vi "License Keya.vi"() -> ()   [LabVIEW 2022 SP3]
panel:
  out "String":string
  in  "Tab Control":enum32{"Page 2"}(tab)
  out "Boolean 4":bool
  out "Boolean 3":bool
  out "Boolean2":bool
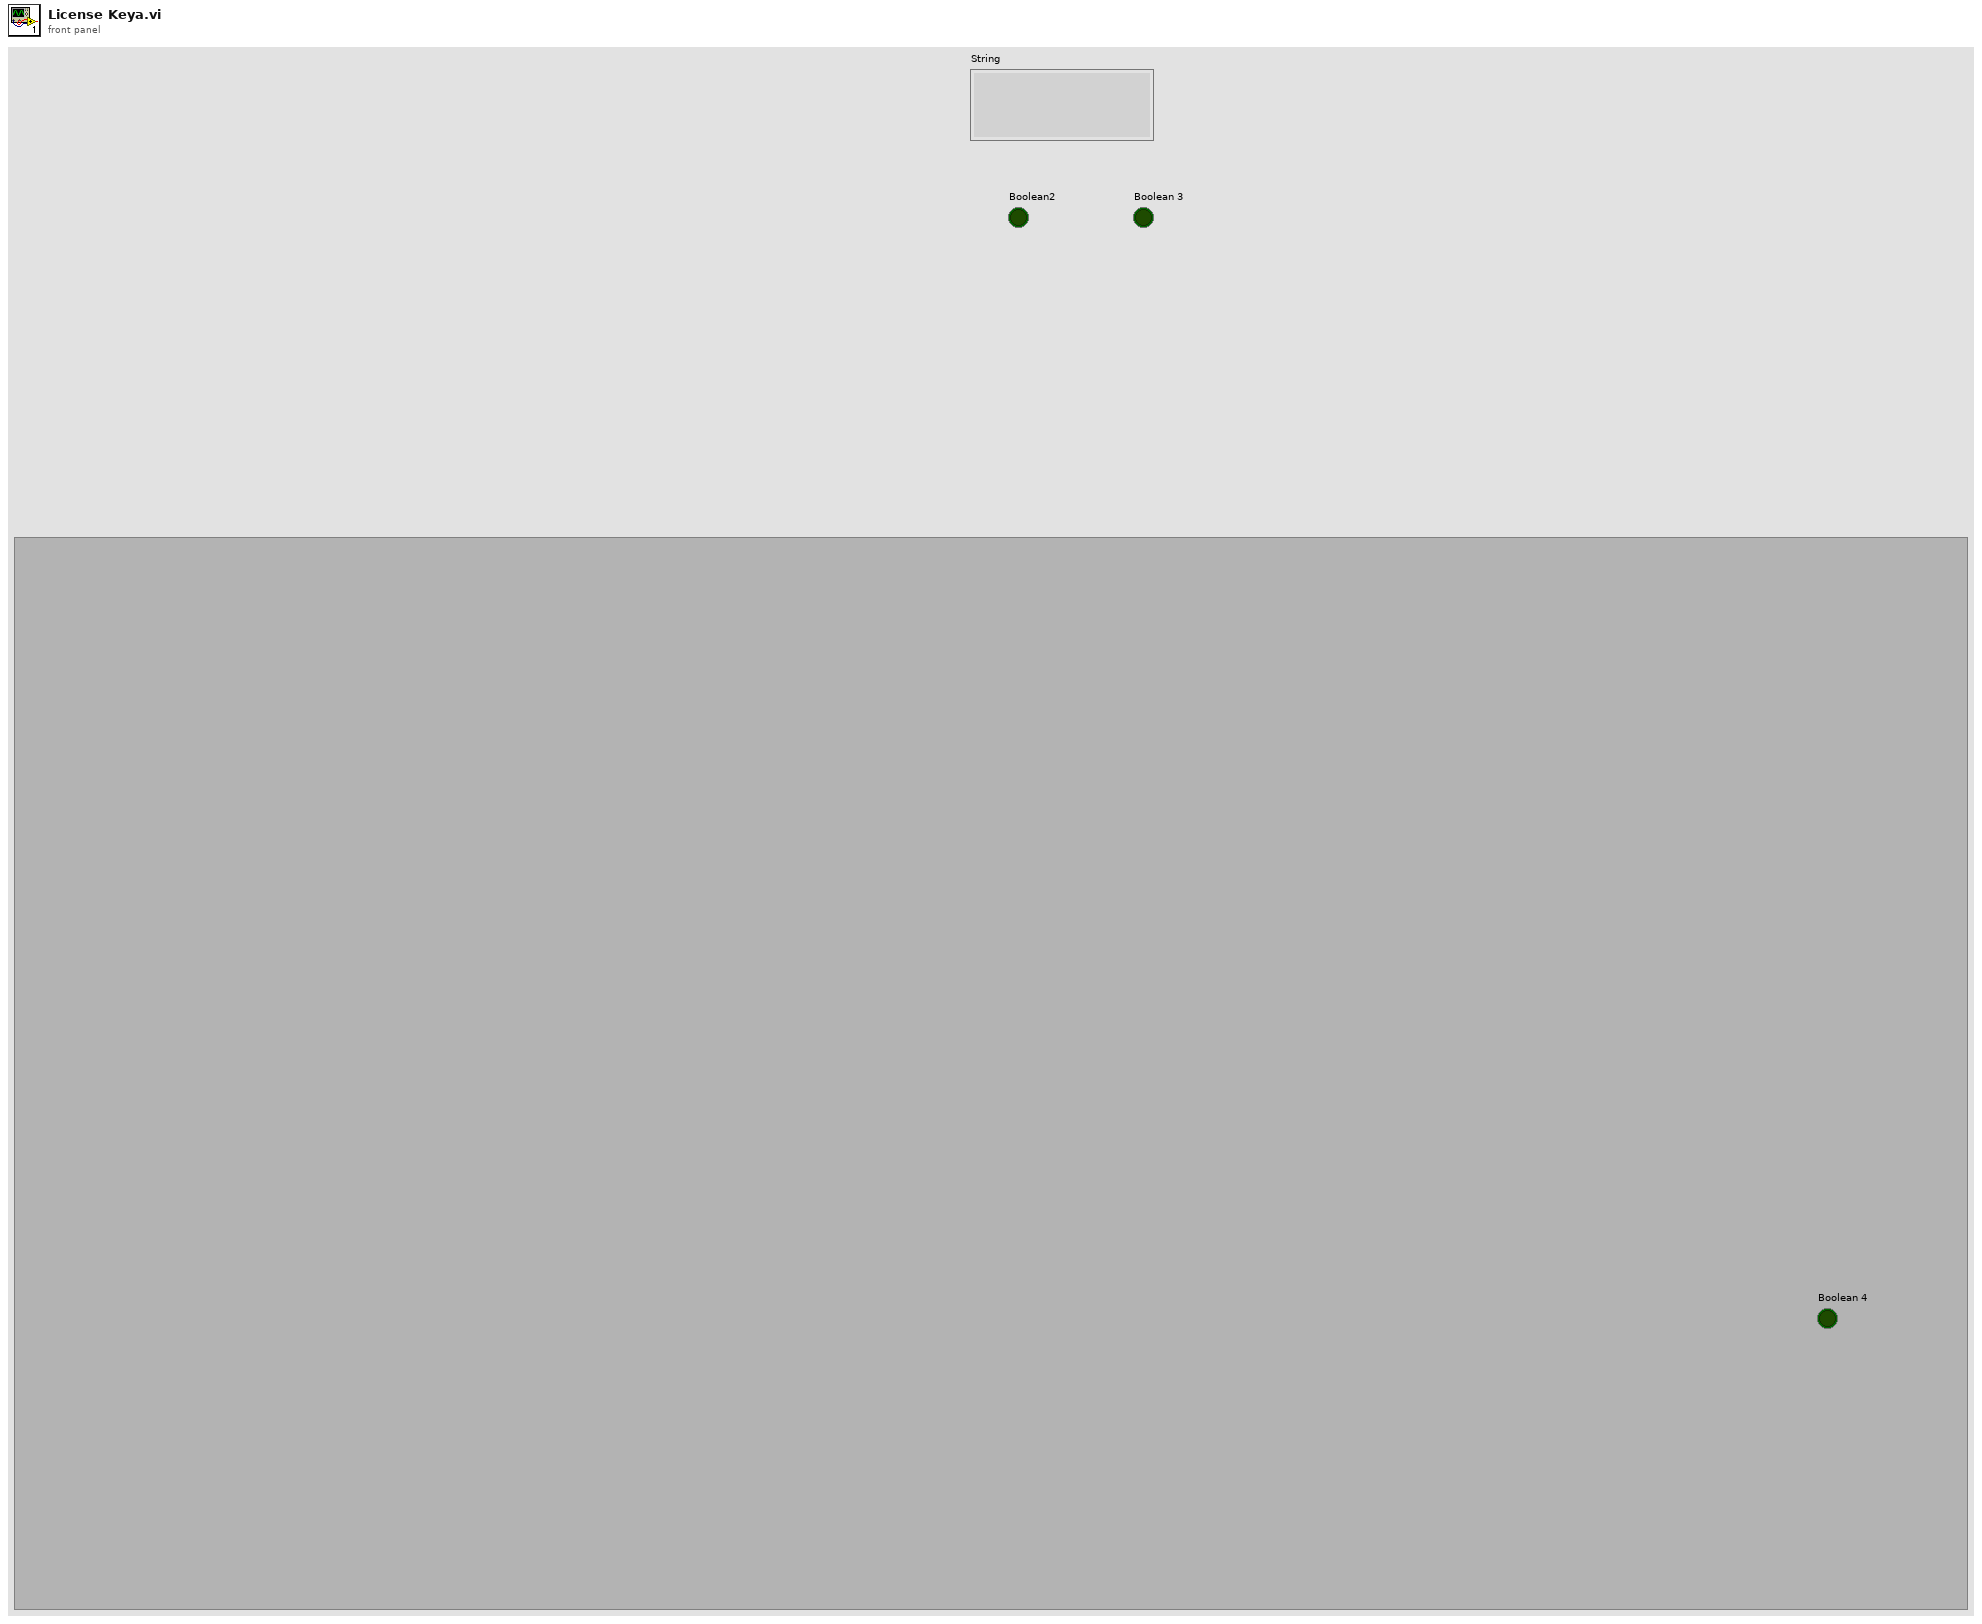
[diagram p1: front panel]
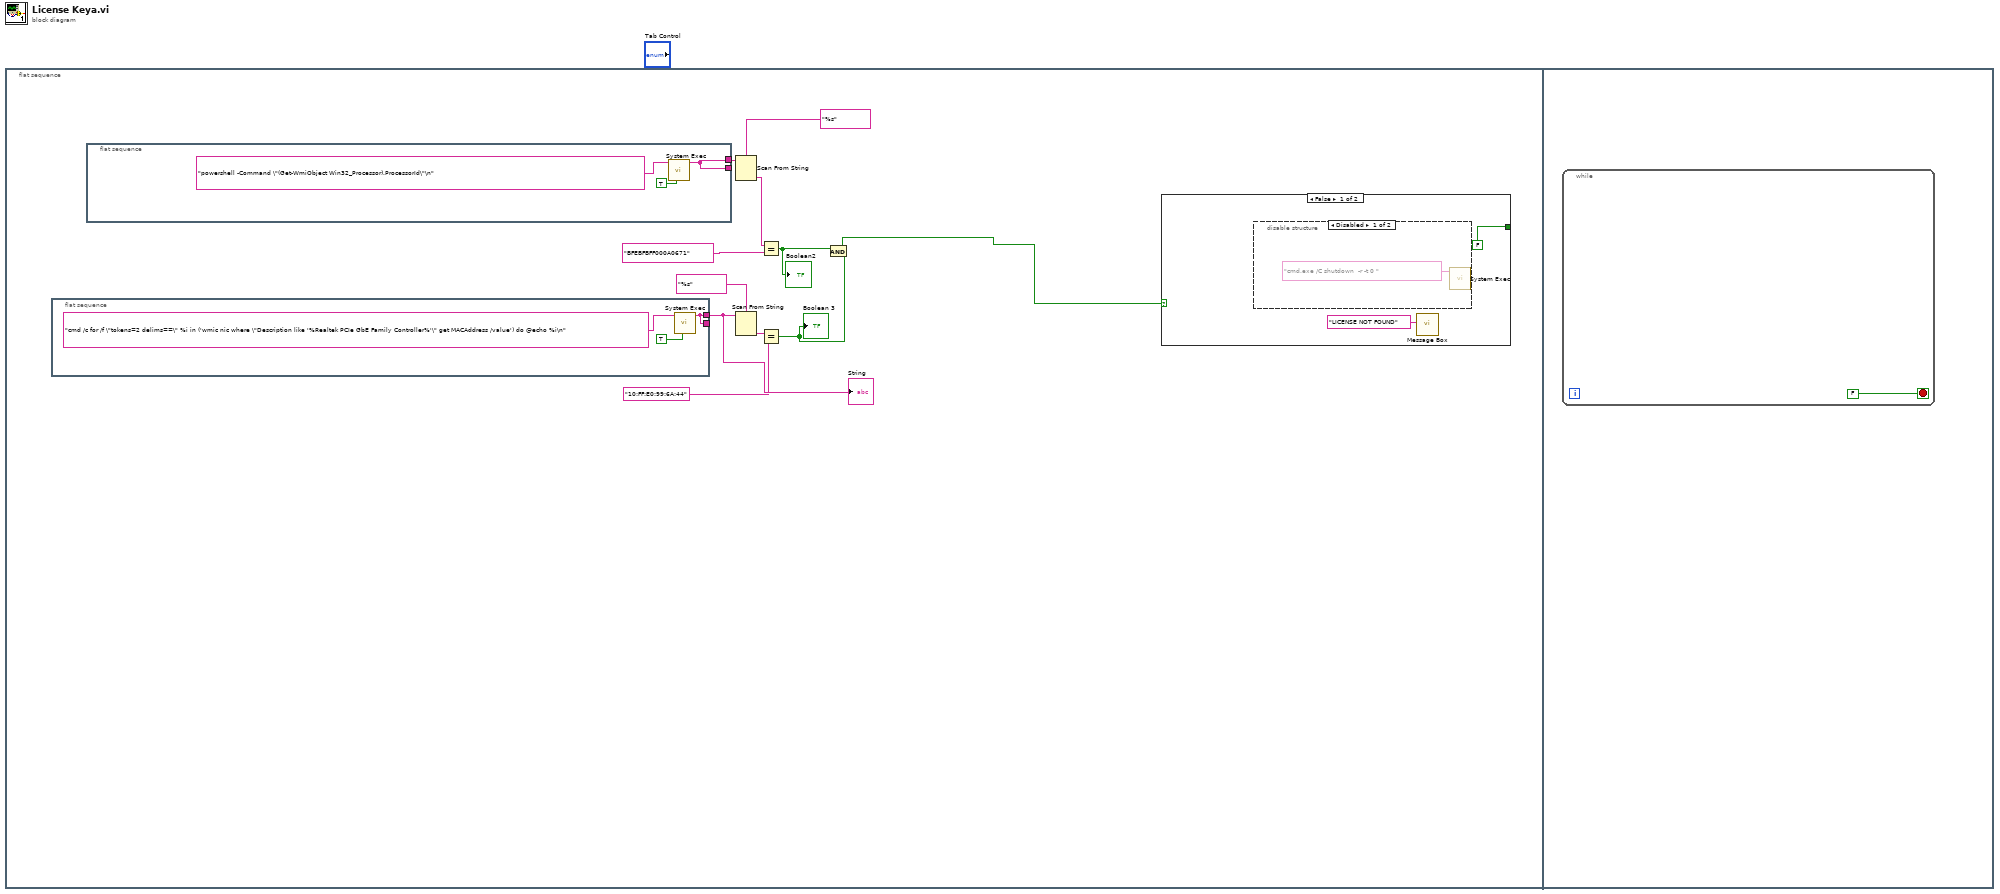
[diagram p0: block diagram]
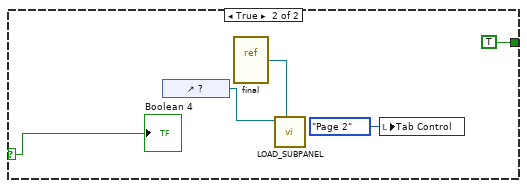
[diagram p3: hidden frame]
diagram:
  n1 = flat-sequence {
    frame #0 {
      n2 = flat-sequence {
        tunnel: [w23] -> w3
        tunnel: [w23] -> _
        frame #0 {
          n3 = call <vilib>:"System Exec.vi"("run minimized? (F)"=TRUE, "command line"="cmd /c for /f \"tokens=2 delims==\" %i in ('wmic nic where \"Description like '%Realtek PCIe GbE Family Controller%'\" get MACAddress /value') do @echo %i\n") -> ("standard output"=w23:string)  [unwired: 6 in, 3 out]
        }
      }
      n4 = flat-sequence {
        tunnel: [w20] -> w7
        tunnel: [w20] -> _
        frame #0 {
          n5 = call <vilib>:"System Exec.vi"("run minimized? (F)"=TRUE, "command line"="powershell -Command \"(Get-WmiObject Win32_Processor).ProcessorId\"\n") -> ("standard output"=w20:string)  [unwired: 6 in, 3 out]
        }
      }
      n6 = Scan From String(format string="%s", input string=w7) -> (output 1=w6:string)  [unwired: 3 in, 3 out]
      n7 = Scan From String(format string="%s", input string=w3) -> (output 1=w9:string)  [unwired: 3 in, 3 out]
      n8 = Equal?(x=w6, y="BFEBFBFF000A0671") -> (x = y?=w5:bool)
      "Boolean2" <- w5
      n9 = Equal?(x=w9, y="10:FF:E0:99:6A:44") -> (x = y?=w4:bool)
      "Boolean 3" <- w4
      n10 = And(x=w5, y=w4) -> (x .and. y?=w1:bool)
      n11 = case shown="False" w1 {
        selector: w1 -> [_ w18]
        tunnel: [FALSE TRUE] -> _
        frame False {
          n12 = disable-structure shown="Disabled" {
            frame Disabled {
              n13 = call <vilib>:"System Exec.vi"("command line"="cmd.exe /C shutdown  -r -t 0 ") -> ()  [unwired: 7 in, 4 out]
            }
            frame Enabled {
            }
          }
          n14 = call "Message Box.vi"("String"="LICENSE NOT FOUND") -> ()  [unwired: 9 in, 1 out]
        }
        frame True {
          n15 = control-ref of="?"() -> (w16:refnum<vi>)
          n16 = vi-ref "final.vi"() -> (w15:refnum<vi>)
          n17 = call "LOAD_SUBPANEL.vi"("SubPanel in"=w16, "VI Ref"=w15) -> ()  [unwired: 8 in, 1 out]
          n18 = local write "Tab Control"(enum32{"Page 2"}."Page 2" ("Tab Control")) -> ()
          "Boolean 4" <- w18
        }
      }
      "String" <- w3
    }
    frame #1 {
      n19 = while {
        stop <- FALSE stop-if-true
      }
    }
  }
